vi "Create Framework Configuration.vi"(8 "error in (no error)":errorcluster, 10 "configuration path":path, 11 "Framework Configuration type":refnum<class "Framework Configuration.lvclass">) -> (0 "error out":errorcluster, 3 "Framework Configuration":refnum<class "Framework Configuration.lvclass">)   [LabVIEW 2017, in "DSF Core.lvlib" / "Framework Configuration.lvclass"]
uses:
  Framework Configuration.lvclass
  Framework Configuration.lvclass/Framework Configuration.ctl
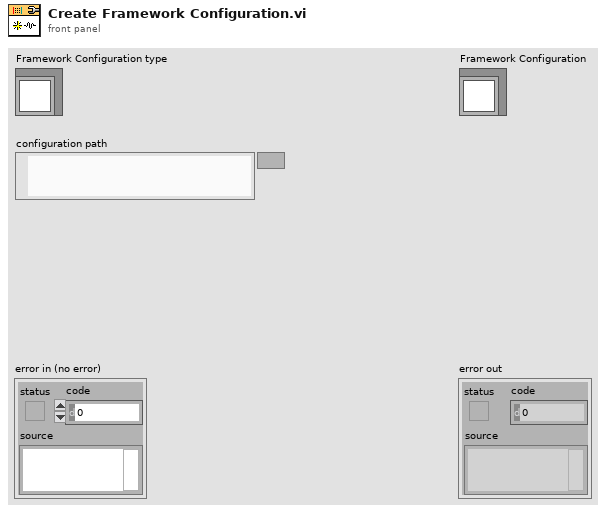
[diagram p1: front panel]
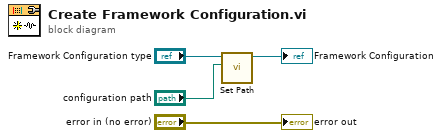
[diagram p0: block diagram]
diagram:
  n1 = call "Set Path.vi"("configuration path"="configuration path", "Framework Configuration in"="Framework Configuration type") -> ("Framework Configuration out"=→"Framework Configuration":refnum<class "Framework Configuration.lvclass">)  [unwired: 9 in]
  "error out" <- "error in (no error)"
